vi "Wind_Tunnel_Main.vi"() -> ()   [LabVIEW 2025]
uses:
  <vilib>/express/express arith-compare/Formula/XNode/ExpressFormulaBlockNode.xnode
  <vilib>/ptbypt/NI_PtbyPt.lvlib
panel:
  out "LC2":dbl
  out "LC0":dbl
  out "LC1":dbl
  in  "CSV-Debug":bool
  out "Voltage Out":dbl
  out "FRQ":dbl
  out "P10(AS1)":dbl
  out "P9":dbl
  out "P8":dbl
  out "P7":dbl
  out "P6":dbl
  out "P5(AS0)":dbl
  out "P4":dbl
  out "P3":dbl
  out "P2":dbl
  out "P1":dbl
  out "Drag":dbl
  in  "Sting Angle":dbl
  out "LC2 Single":dbl
  out "LC1 Single":dbl
  out "LC0 Single":dbl
  in  "Spreadsheet Path":path=path "C:/Users/student/Desktop/Wind Tunnel Software/Testing Data"
  out "Lift?":dbl
  out "Estimated Velocity":dbl
  in  "Single Shot":bool
  in  "Spreadsheet Name. (Needs to end in \".csv\")":string="%Y-%m-%d_%H-%M-%S.csv"
  out "ESTOP ACTIVE":bool
  in  "ESTOP":bool
  in  "SYSTEM TARE":bool
  in  "Tare LC0":bool
  out "?":dbl
  out "LC0":dbl(graph)
  in  "Tare LC1":bool
  out "?":dbl
  out "LC1":dbl(graph)
  in  "Tare LC2":bool
  in  "Tare Pitot Tube\nNote: ONLY USE AT\nIDLE":bool
  out "?":dbl
  out "LC2":dbl(graph)
  out "?":bool
  out "?":bool
  in  "VFD \nMode\nSelect":bool=TRUE
  out "VFD Frequency":dbl
  in  "Speed %\n0-100":dbl
  in  "Target Speed (m/s)":dbl
  out "V_DIFF":dbl
  out "Dynamic Voltage":dbl format="%0.2f"
  out "Static Voltage":dbl format="%0.2f"
  in  "Enable Data Collection\n(Excel Spreadsheet)":bool caption="Enable"
  out "?":bool
  out "Airspeed Warning Indicator":string
  out "IAS (m/s)":dbl format="%#_4g"
  out "Indicated Velocity Graph (m/s)":dbl(graph)
  in  "System Stop":bool=TRUE
  # "System Controls"
  # "Wind Tunnel Data"
  # "Quick Start"
  # "Raw Voltage Data"
  # "0. Read the Documentation!!!\n1. Familiarize yourself with this panel. Pressing Ctrl+H will bring up a help menu. Clicking components will bring up more information.\n2.Looking at the graphs, they will not be zeroed\nTo fix this press SYSTEM TARE (bottom right of this Panel).  You should expect the graphs to the right to be within +- 5 of zero after tare. \n3. Looking at the VFD box (the one attached to \nthe fan with dials/switches) make sure it is set\nto ON, switched to Automated, and check that the Emergency Stop button is not pressed. If it is, twist it clockwise to reset"
  # "4. Now the fan is controlled by this panel. On the\n\"Fan Controls\" below, set the \"VFD mode switch\" to the upward postition to to enable Speed % Mode, which controls the fan by a percentage of its maximum power. You can now adjust the box \"Speed %\" which will spin up the fan.\n\nNOTE:  To save data to CSV, first hit \"System Stop\", then refer to the controls on the bottom of this panel. Select the Enable Data Collection button so it displays \"Enabled\". Then set the Spreadsheet Path by selecting the little folder icon and following the prompts. Change the name as desired. Start over from step 0"
  # "Pitot Tube\nControls"
  # "Shutdown Procedure"
  # "Fan Controls"
  # "1. Set both speed % and target speed controls to 0. Wait for fan to spin down\n2. Press system stop.\n3. On the VFD, set the switch to \"MANUAL\", press the physical E-Stop, make sure dial is set to 0, and then set the switch to \"OFF \".\n4. Set the switch on the power box to the downward off position and lock.\n5. Unplug the black powerstrip behind this computer"
  # "Measurements inaccurate under 10m/s"
  # "MAX 100"
  # "MAX 70"
  # "System Controls"
  # "Derived Values:"
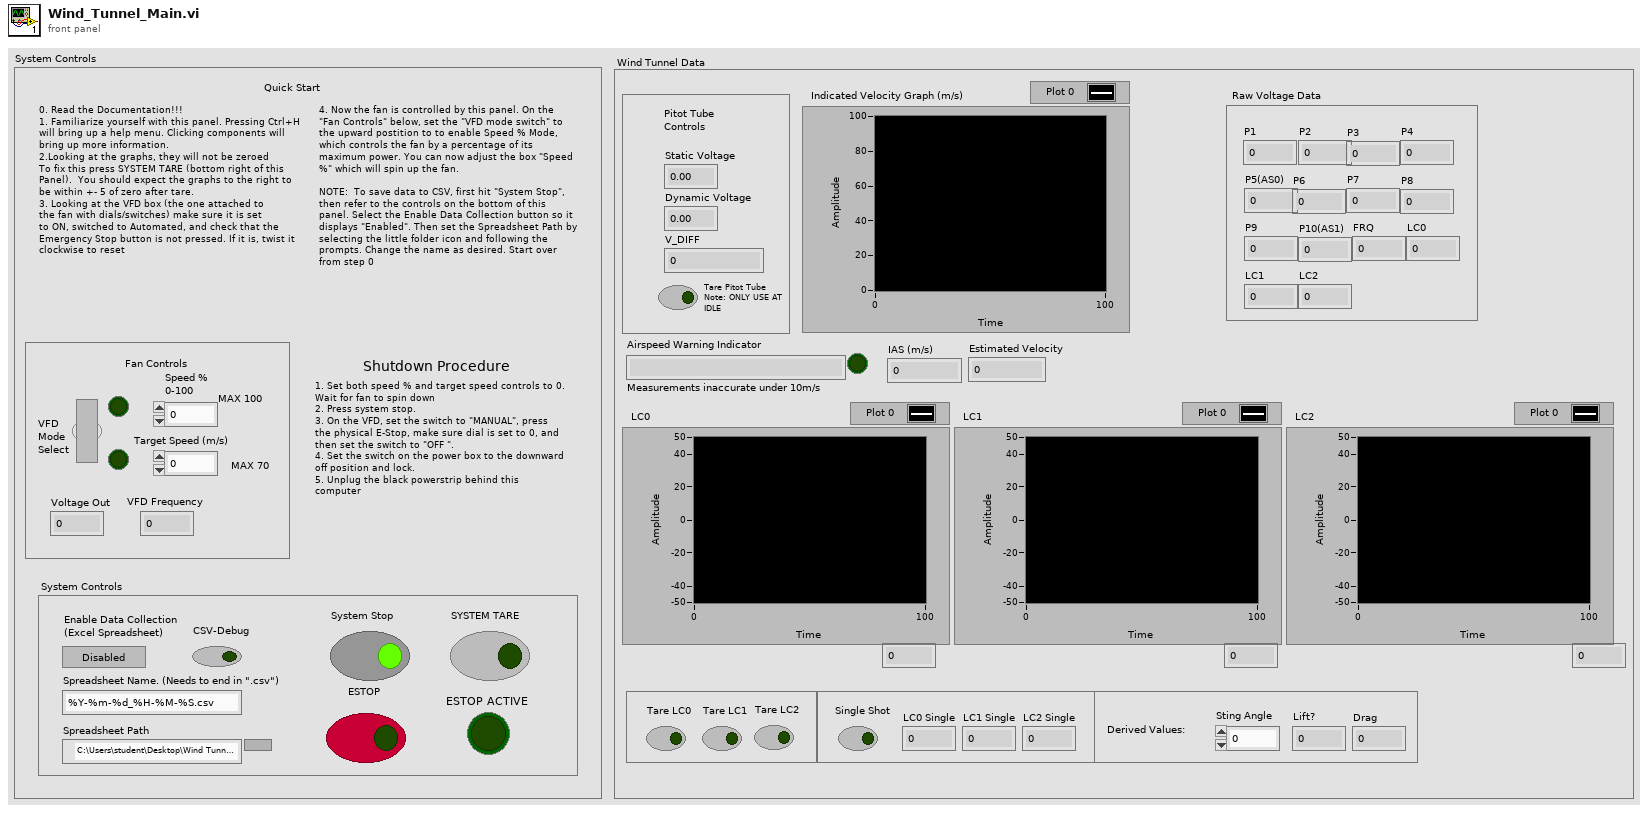
[diagram p1: front panel]
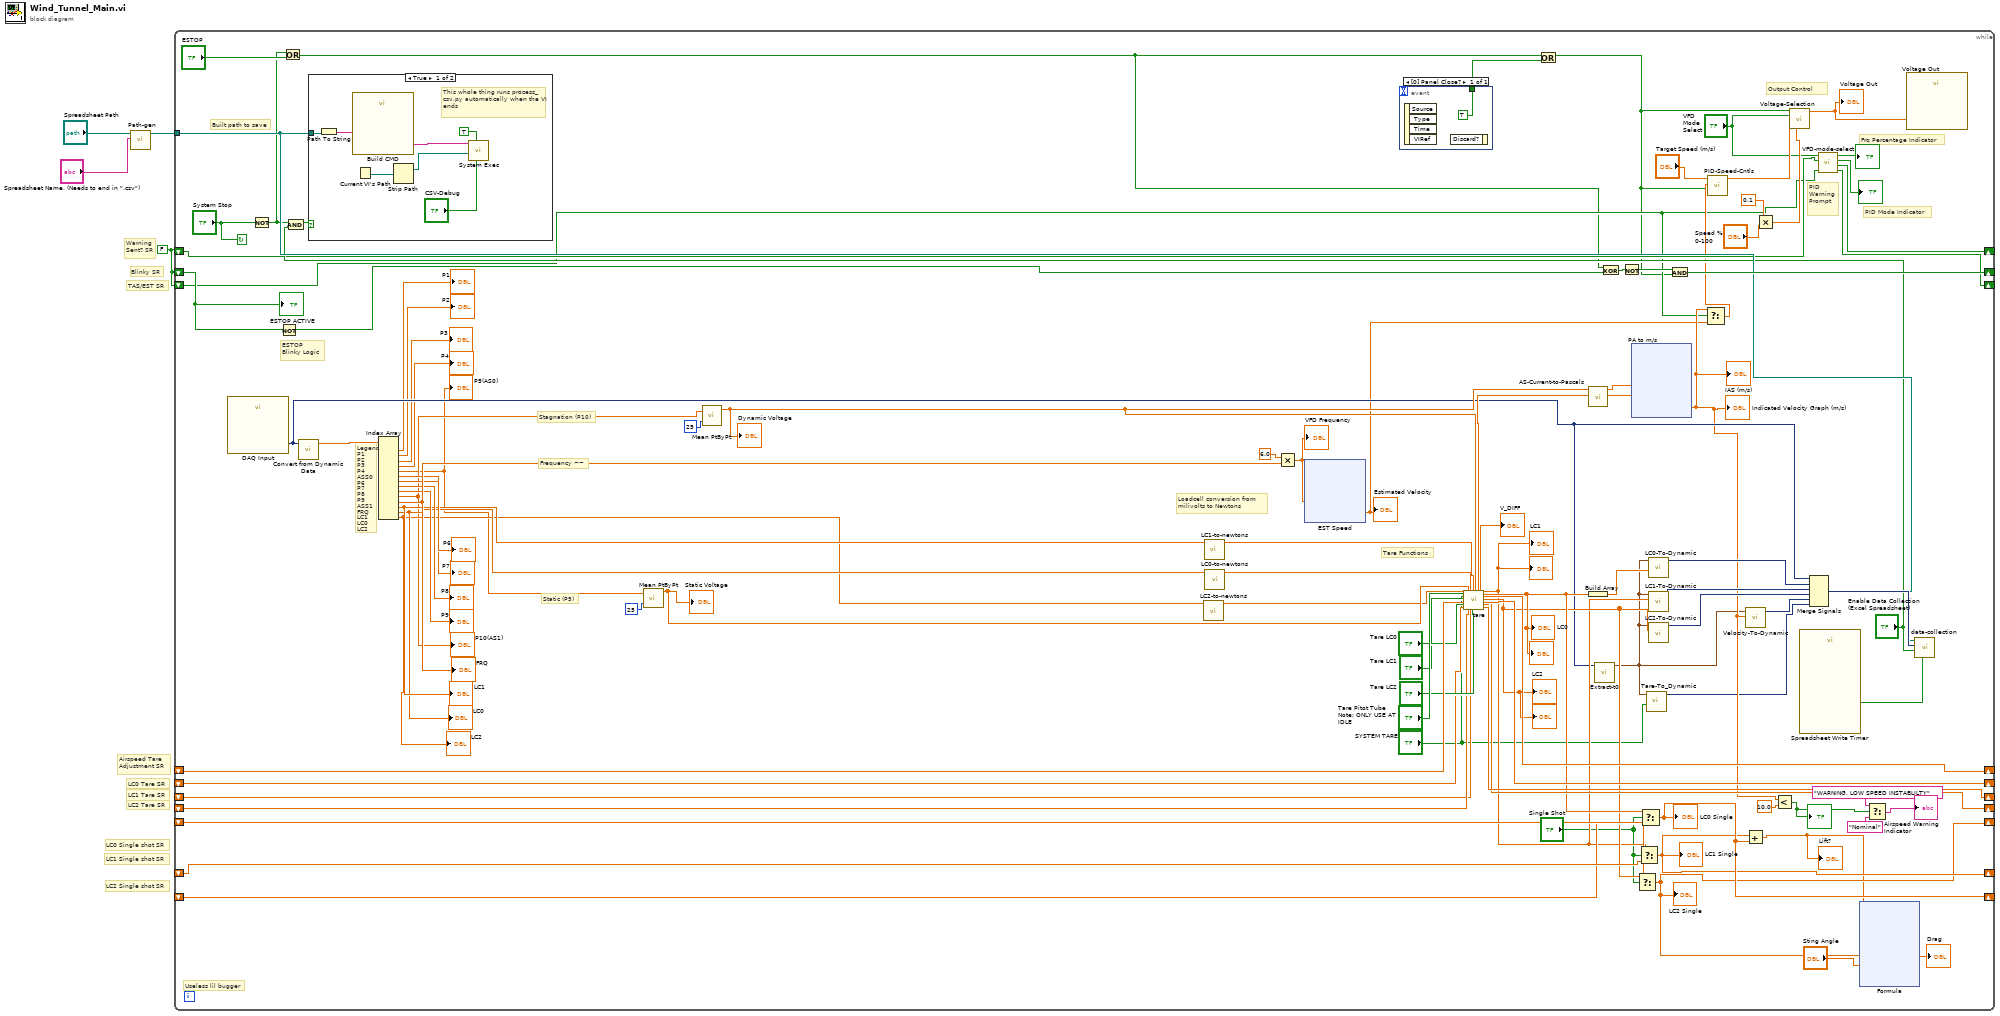
[diagram p0: block diagram]
diagram:
  w1 = FALSE
  # "TAS/EST SR"
  # "LC2 Tare SR"
  # "LC2 Single shot SR"
  # "LC1 Single shot SR"
  # "LC0 Single shot SR"
  # "LC1 Tare SR"
  # "LC0 Tare SR"
  # "Airspeed Tare\nAdjustment SR"
  # "Warning\nSent? SR"
  # "Blinky SR"
  n1 = call "Path-gen.vi"("Spreadsheet Name"="Spreadsheet Name. (Needs to end in \".csv\")", "Spreadsheet Path"="Spreadsheet Path") -> ("appended path"=w4:path)  [unwired: 9 in]
  n2 = while {
    tunnel: w4 -> [w35]
    shift-right: [w90] -> _
    shift-left: _ -> [w91]
    shift-right: [w77] -> _
    shift-left: _ -> [w86]
    shift-right: [w81] -> _
    shift-left: _ -> [w87]
    shift-right: [w79] -> _
    shift-left: _ -> [w42]
    shift-right: [w72] -> _
    shift-left: w1 -> [w74]
    shift-right: [w23] -> _
    shift-left: w1 -> [w26]
    shift-right: [w56] -> _
    shift-left: _ -> [w68]
    shift-right: [w55] -> _
    shift-left: _ -> [w70]
    shift-right: [w54] -> _
    shift-left: _ -> [w69]
    shift-right: [w22] -> _
    shift-left: w1 -> [w19]
    stop <- "System Stop" continue-if-true
    # "Loadcell conversion from\nmilivolts to Newtons"
    # "Tare Functions"
    # "Built path to save"
    # "Useless lil bugger"
    # "Frequency ~~"
    # "Static (P5)"
    # "Stagnation (P10)"
    # "ESTOP\nBlinky Logic"
    # "Frq Percentage Indicator"
    # "PID Mode Indicator"
    # "PID \nWarning\nPrompt"
    # "Output Control"
    # "Legend\nP1\nP2\nP3\nP4\nASS0\nP6\nP7\nP8\nP9\nASS1\nFRQ\nLC1\nLC0\nLC2"
    n3 = call "DAQ Input"() -> ("data"=w58:dynamicdata)  [unwired: 16 in, 3 out]
    n4 = Not(x="System Stop") -> (.not. x?=w15:bool)
    n5 = Not(x=w74) -> (.not. x?=w73:bool)
    n6 = Or(x=w15, y="ESTOP") -> (x .or. y?=w16:bool)
    n7 = And(x=w15, y="Enable Data Collection\n(Excel Spreadsheet)") -> (x .and. y?=w29:bool)
    n8 = call "Convert from Dynamic Data"("Dynamic Data Type"=w58) -> ("Array"=w103:dbl[])  [unwired: 3 in]
    n9 = case shown="True" w29 {
      tunnel: w35 -> [w123 _]
      frame True {
        # "This whole thing runs process_csv.py automatically when the VI ends"
        n10 = Path To String(path=w123) -> (string=w122:string)
        n11 = call "Build CMD"("s"=w122) -> ("Result"=w121:string)  [unwired: 13 in, 1 out]
        n12 = Current VI's Path() -> (path=w119:path)
        n13 = Strip Path(path=w119) -> (stripped path=w118:path)  [unwired: 1 out]
        n14 = call <vilib>:"System Exec.vi"("run minimized? (F)"="CSV-Debug", "wait until completion? (T)"=TRUE, "working directory"=w118, "command line"=w121) -> ()  [unwired: 4 in, 4 out]
      }
      frame False {
      }
    }
    n15 = Index Array(array=w103) -> (element #1=→"P1":dbl, element #2=→"P2":dbl, element #3=→"P3":dbl, element #4=→"P4":dbl, element #5=w37:dbl, element #6=→"P6":dbl, element #7=→"P7":dbl, element #8=→"P8":dbl, element #9=→"P9":dbl, element #10=w38:dbl, element #11=w92:dbl, element #12=w41:dbl, element #13=w40:dbl, element #14=w39:dbl)  [unwired: 14 in]
    "P5(AS0)" <- w37
    "P10(AS1)" <- w38
    "FRQ" <- w92
    "LC1" <- w41
    "LC0" <- w40
    "LC2" <- w39
    n16 = call <vilib>:"Mean PtByPt.vi"("x"=w37, "sample length"=25) -> ("mean"=w100:dbl)  [unwired: 2 in, 1 out]
    "Static Voltage" <- w100
    n17 = call <vilib>:"Mean PtByPt.vi"("x"=w38, "sample length"=25) -> ("mean"=w99:dbl)  [unwired: 2 in, 1 out]
    "Dynamic Voltage" <- w99
    n18 = call "LC2-to-newtons.vi"("mv in"=w39) -> ("newtons out"=w76:dbl)  [unwired: 10 in]
    n19 = call "LC1-to-newtons.vi"("LC In"=w41) -> ("Newtons Out"=w80:dbl)  [unwired: 10 in]
    n20 = call "LC0-to-newtons.vi"("mv in"=w40) -> ("newtons out"=w78:dbl)  [unwired: 10 in]
    n21 = Multiply(x=6.0, y=w92) -> (x*y=w57:dbl)
    "VFD Frequency" <- w57
    n22 = xnode "EST Speed"("X1"=w57) -> ("Result"=w18:dbl)  [unwired: 1 in, 1 out]
    "Estimated Velocity" <- w18
    n23 = event shown="[0] Panel Close?" {
      selector: _ -> [_]
      dyn-events: _ -> [_]
      timeout: _ -> [_]
      tunnel: [TRUE] -> w5
      event Panel Close? {
        n24 = event-data() -> ()  [unwired: 1 in, 4 out]
        n25 = event-data() -> ()  [unwired: 2 in, 1 out]
      }
    }
    n26 = call "tare.vi"("LC2 Tare\nAmount"=w76, "Tare Pitot Tube\nNote: ONLY USE AT\nIDLE"="Tare Pitot Tube\nNote: ONLY USE AT\nIDLE", "SYSTEM TARE\nONLY USE AT IDLE"="SYSTEM TARE", "Tare LC1"="Tare LC1", "Previous \nAdjustment"=w91, "Tare LC0"="Tare LC0", "LC0 Prev"=w87, "AS 0"=w100, "LC2 Prev"=w86, "LC1 Tare \nAmount"=w78, "LC1 Prev"=w42, "LC0 Tare\nAmount"=w80, "Tare LC2"="Tare LC2", "AS 1"=w99) -> ("AS0 Out"=w98:dbl, "V_DIFF\nIndicator"=→"V_DIFF":dbl, "LC1 Out"=w64:dbl, "LC0 Out"=w66:dbl, "Adjustment To Shift"=w90:dbl, "LC2 Out"=w65:dbl, "LC0 To\nShift"=w81:dbl, "LC2 To \nShift"=w77:dbl, "LC1 to \nShift"=w79:dbl)  [unwired: 5 in]
    "LC2" <- w65
    "?" <- w65
    "LC1" <- w64
    "?" <- w64
    "LC0" <- w66
    "?" <- w66
    n27 = Or(x=w16, y=w5) -> (x .or. y?=w6:bool)
    n28 = call "AS-Current-to-Pascals.vi"("V0 In"=w98, "V1 In"=w99) -> ("PA1 Out"=w102:dbl, "PA0 Out"=w96:dbl)  [unwired: 8 in]
    n29 = Build Array(w66) -> (w62:dbl[])
    n30 = call "Extract-t0.vi"("data"=w58) -> ("Waveform"=w14:waveform(dbl))  [unwired: 10 in]
    n31 = Exclusive Or(1:w73, 2:w16) -> (0:w75:bool)
    n32 = Not(x=w75) -> (.not. x?=w71:bool)
    n33 = xnode ("PA to m/s")("pa0"=w96, "pa1"=w102) -> ("Result"=w21:dbl)  [unwired: 1 in, 1 out]
    "Indicated Velocity Graph (m/s)" <- w21
    "IAS (m/s)" <- w21
    n34 = Select(t=w65, s="Single Shot", f=w69) -> (s? t:f=w54:dbl)
    "LC2 Single" <- w54
    n35 = Select(t=w64, s="Single Shot", f=w70) -> (s? t:f=w55:dbl)
    "LC1 Single" <- w55
    n36 = Select(t=w66, s="Single Shot", f=w68) -> (s? t:f=w56:dbl)
    "LC0 Single" <- w56
    n37 = call "Tare-To_Dynamic.vi"("Tare In"="SYSTEM TARE", "Waveform"=w14) -> ("Dynamic Data Type"=w12:dynamicdata)  [unwired: 9 in]
    n38 = call "LC0-To-Dynamic.vi"("Array"=w62, "Waveform"=w14) -> ("Dynamic Data Type"=w61:dynamicdata)  [unwired: 9 in]
    n39 = call "LC1-To-Dynamic.vi"("Numeric"=w64, "Waveform"=w14) -> ("Dynamic Data Type"=w59:dynamicdata)  [unwired: 9 in]
    n40 = call "LC2-To-Dynamic.vi"("Numeric"=w65, "Waveform"=w14) -> ("Dynamic Data Type"=w60:dynamicdata)  [unwired: 9 in]
    n41 = And(x=w71, y=w6) -> (x .and. y?=w72:bool)
    n42 = Select(t=w21, s=w19, f=w18) -> (s? t:f=w20:dbl)
    n43 = call "PID-Speed-Cntls.vi"("ESTOP"=w6, "PID IN"=w20, "Target Speed (m/s)"="Target Speed (m/s)") -> ("output"=w33:dbl)  [unwired: 8 in]
    n44 = call "Velocity-To-Dynamic.vi"("Result"=w21, "Waveform"=w14) -> ("Dynamic Data Type"=w63:dynamicdata)  [unwired: 9 in]
    n45 = Add(x=w55, y=w56) -> (x+y=w11:dbl)
    "Lift?" <- w11
    n46 = Multiply(x=0.1, y="Speed %\n0-100") -> (x*y=w32:dbl)
    n47 = Less?(x=w21, y=10.0) -> (x < y?=w8:bool)
    "?" <- w8
    n48 = call "Voltage-Selection.vi"("ESTOP"=w6, "VFD \nMode\nSelect"="VFD \nMode\nSelect", "PID In"=w33, "Percentage\nIn"=w32) -> ("output"=w30:dbl)  [unwired: 11 in]
    "Voltage Out" <- w30
    n49 = call "Spreadsheet Write Timer"() -> ("Time has Elapsed"=w97:bool)  [unwired: 12 in, 7 out]
    n50 = Merge Signals(w58, w61, w59, w60, w63, w12) -> (w67:dynamicdata)
    n51 = call "VFD-mode-select.vi"("Est/TAS IN"=w19, "Warning\nSent? IN"=w26, "VFD \nMode\nSelect"="VFD \nMode\nSelect") -> ("EST/TAS out"=w22:bool, "Warning\nSent? OUT"=w23:bool, "PID Mode Indc"=→"?":bool, "FRQ Indc"=→"?":bool)  [unwired: 5 in]
    n52 = xnode "Formula"("L"=w11, "LC2"=w54, "theta"="Sting Angle") -> ("Result"=→"Drag":dbl)  [unwired: 1 in, 1 out]
    n53 = Select(t="WARNING. LOW SPEED INSTABLILTY", s=w8, f="Nominal") -> (s? t:f=→"Airspeed Warning Indicator":string)
    n54 = call "Voltage Out"("data"=w30) -> ()  [unwired: 17 in, 2 out]
    n55 = call "data-collection.vi"("Time has Elapsed"=w97, "Enable Data Collection\n(Excel Spreadsheet)"="Enable Data Collection\n(Excel Spreadsheet)", "Dynamic Data"=w67, "appended path"=w35) -> ()  [unwired: 8 in]
    "ESTOP ACTIVE" <- w74
  }
